vi "Center Loading Cluster Elements.vi"(8 "error in (no error)":errorcluster, 10 "string/path":string, 11 "Cluster in":refnum<vi>) -> (0 "error out":errorcluster)   [LabVIEW 2014]
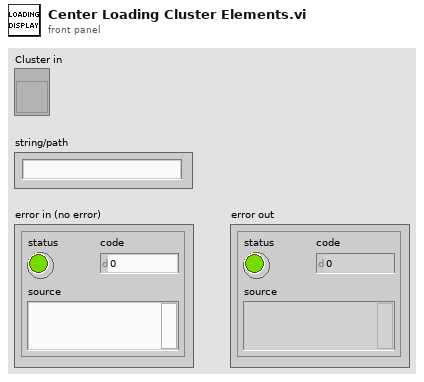
[diagram p1: front panel]
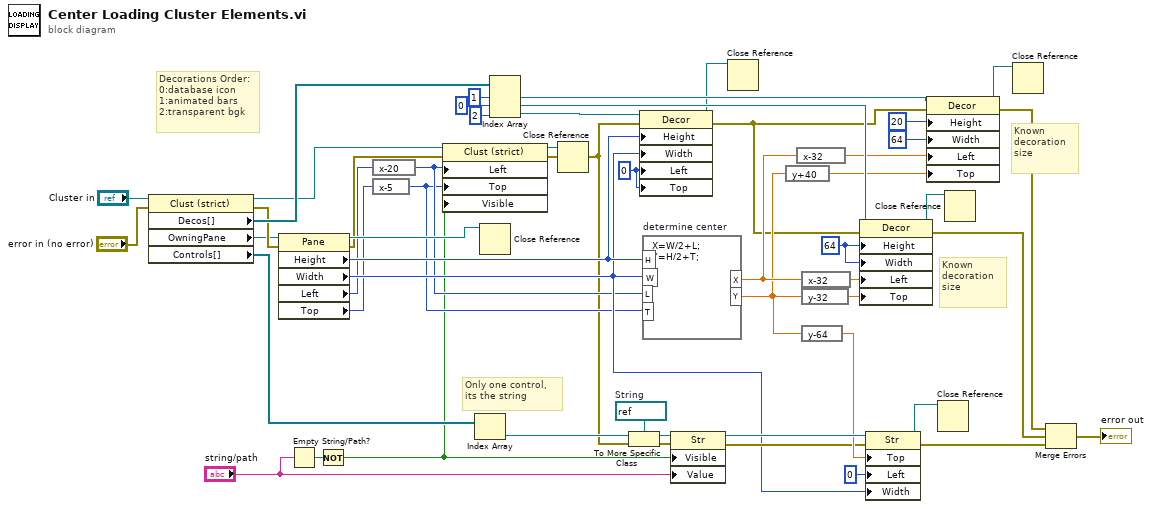
[diagram p0: block diagram]
diagram:
  w5 = 0 ("Position:Left")
  w44 = u32 64 ("Size:Height")
  w49 = refnum<vi> refnum  # String
  # "Only one control, its the string"
  # "Known decoration size"
  # "Known decoration size"
  # "Decorations Order:\n0:database icon\n1:animated bars\n2:transparent bgk"
  n1 = property class="Clust (strict)"(reference="Cluster in", error in="error in (no error)") -> (reference out=w11:refnum<vi>, error out=w28:errorcluster, "Decos[]"=w52:refnum<vi>[], "OwningPane"=w12:refnum<vi>, "Controls[]"=w15:refnum<vi>[])
  n2 = property class="Pane"(reference=w12, error in=w28) -> (reference out=w16:refnum<vi>, error out=w3:errorcluster, "Height"=w14:u32, "Width"=w13:u32, "Left"=w8:i32, "Top"=w9:i32)
  n3 = Empty String/Path?(string/path="string/path") -> (empty?=w51:bool)
  n4 = Not(x=w51) -> (.not. x?=w1:bool)
  n5 = expression code="x-20"(w8) -> (w7:i32)
  n6 = expression code="x-5"(w9) -> (w6:i32)
  n7 = property class="Clust (strict)"(reference=w11, error in=w3, "Left"=w7, "Top"=w6, "Visible"=w1) -> (reference out=w10:refnum<vi>, error out=w2:errorcluster)
  n8 = Index Array(array=w15) -> (element=w47:refnum<vi>)  [unwired: 1 in]
  n9 = Close Reference(reference=w16) -> ()  [unwired: 1 in, 1 out]
  n10 = Index Array(array=w52, index #1=1 ("index"), index #2=0 ("index"), index #3=2 ("index")) -> (element #1=w38:refnum<vi>, element #2=w45:refnum<vi>, element #3=w53:refnum<vi>)
  n11 = Close Reference(reference=w10) -> ()  [unwired: 1 in, 1 out]
  n12 = To More Specific Class(target class=w49, reference=w47, error in=w2) -> (specific class reference=w48:refnum<vi>, error out=w26:errorcluster)
  n13 = property class="Decor"(reference=w53, error in=w2, "Height"=w14, "Width"=w13, "Left"=w5, "Top"=w5) -> (reference out=w17:refnum<vi>, error out=w27:errorcluster)
  n14 = formula code="X=W/2+L;\nY=H/2+T;" "determine center"("H"=w14, "W"=w13, "L"=w7, "T"=w6) -> ("X"=w37:dbl, "Y"=w35:dbl)
  n15 = property class="Str"(reference=w48, error in=w26, "Visible"=w1, "Value"="string/path") -> (reference out=w36:refnum<vi>, error out=w25:errorcluster)
  n16 = Close Reference(reference=w17) -> ()  [unwired: 1 in, 1 out]
  n17 = expression code="y+40"(w35) -> (w41:dbl)
  n18 = expression code="x-32"(w37) -> (w40:dbl)
  n19 = expression code="x-32"(w37) -> (w43:dbl)
  n20 = expression code="y-32"(w35) -> (w42:dbl)
  n21 = expression code="y-64"(w35) -> (w34:dbl)
  n22 = property class="Decor"(reference=w45, error in=w27, "Height"=w44, "Width"=w44, "Left"=w43, "Top"=w42) -> (reference out=w19:refnum<vi>, error out=w23:errorcluster)
  n23 = property class="Str"(reference=w36, error in=w25, "Top"=w34, "Left"=0 ("Position:Left"), "Width"=w13) -> (reference out=w20:refnum<vi>, error out=w22:errorcluster)
  n24 = property class="Decor"(reference=w38, error in=w27, "Height"=u32 20 ("Size:Height"), "Width"=u32 64 ("Size:Height"), "Left"=w40, "Top"=w41) -> (reference out=w18:refnum<vi>, error out=w24:errorcluster)
  n25 = Close Reference(reference=w20) -> ()  [unwired: 1 in, 1 out]
  n26 = Close Reference(reference=w19) -> ()  [unwired: 1 in, 1 out]
  n27 = Close Reference(reference=w18) -> ()  [unwired: 1 in, 1 out]
  n28 = Merge Errors(w24, w23, w22) -> (→"error out":errorcluster)
